vi "14_StartStop_UI.vi"(8 "error in (no error)":errorcluster) -> (0 "error out":errorcluster)   [LabVIEW 2014]
uses:
  SwabianInstruments.TimeTagger
panel:
  in  "clear":bool
  in  "binwidth":i64=1
  in  "Test signal":bool
  in  "Start channel":i32=2
  in  "Stop channel":i32=1
  in  "stop":bool
  out "StartStop Histogram":cluster{i64[], i64[]}(graph)
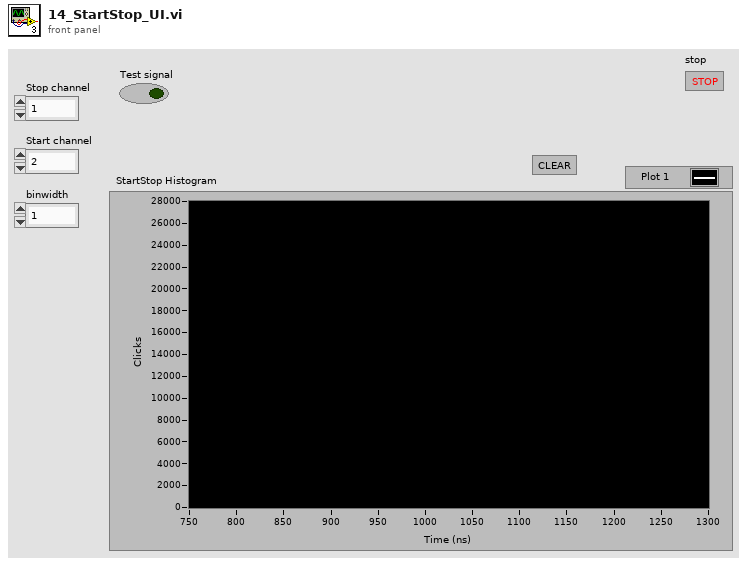
[diagram p1: front panel]
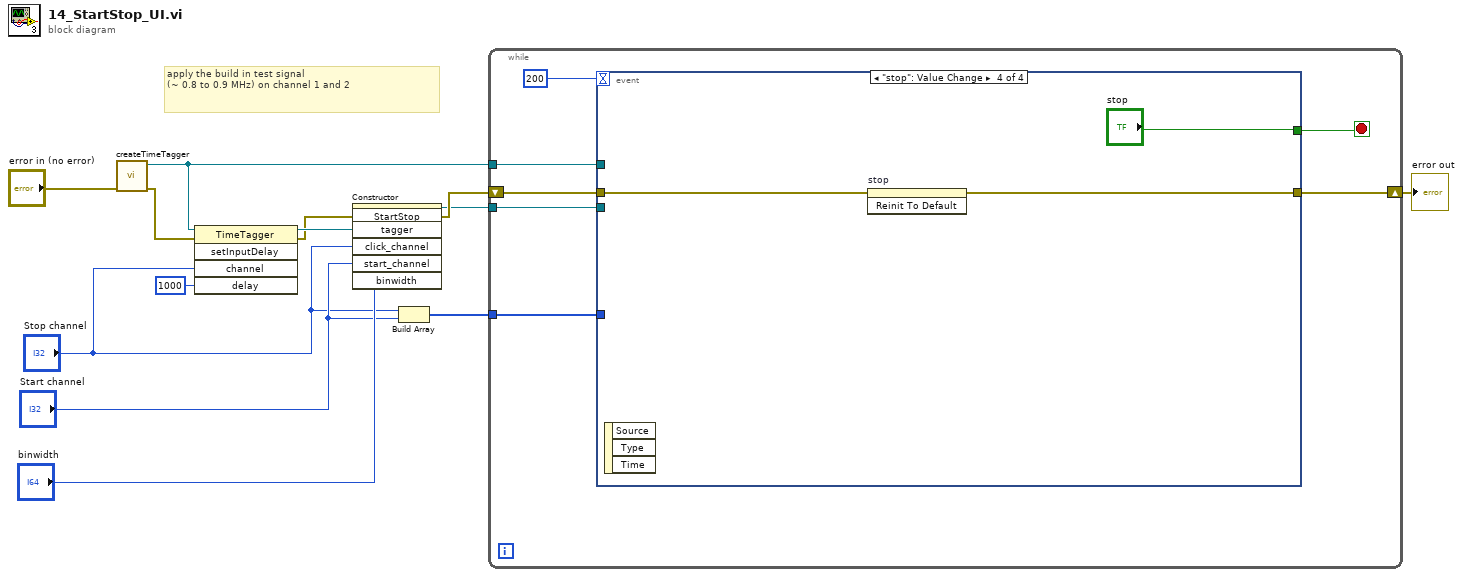
[diagram p0: block diagram]
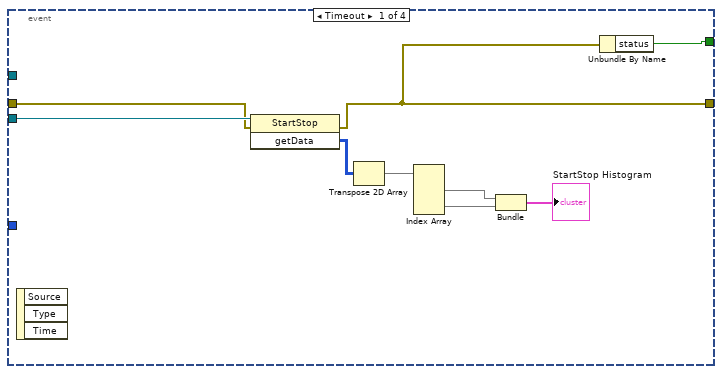
[diagram p2: hidden frame]
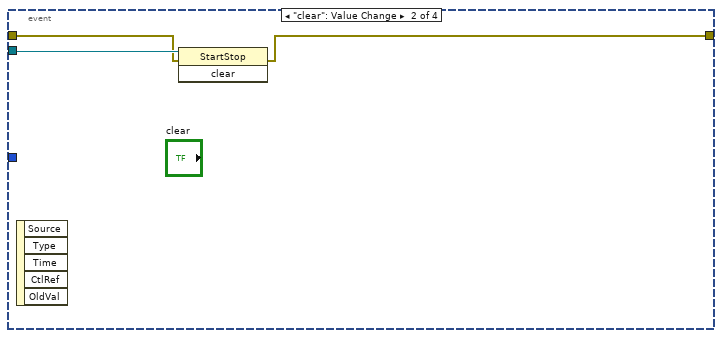
[diagram p3: hidden frame]
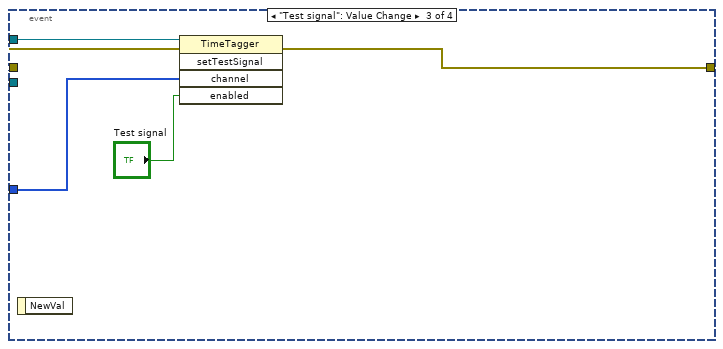
[diagram p4: hidden frame]
diagram:
  # "apply the build in test signal\n(~ 0.8 to 0.9 MHz) on channel 1 and 2"
  n1 = call "createTimeTagger.vi"("error in (no error)"="error in (no error)") -> ("error out"=w3:errorcluster, "TimeTagger ref out"=w6:refnum<k24>)  [unwired: 9 in]
  n2 = invoke class="TimeTagger" method="setInputDelay"(reference=w6, error in=w3, "channel"="Stop channel", "delay"=i64 1000) -> (reference out=w5:refnum<k24>, error out=w2:errorcluster)  [unwired: 1 in, 3 out]
  n3 = constructor class="StartStop"(error in=w2, "tagger"=w5, "click_channel"="Stop channel", "start_channel"="Start channel", "binwidth"="binwidth") -> (reference out=w12:refnum<k24>, error out=w13:errorcluster)  [unwired: 2 in, 5 out]
  n4 = Build Array("Stop channel", "Start channel") -> (w9:i32[])
  n5 = while {
    tunnel: w6 -> [w19]
    shift-right: [w18] -> w7
    shift-left: w13 -> [w20]
    tunnel: w12 -> [w17]
    tunnel: w9 -> [w15]
    stop <- w14 stop-if-true
    n6 = event shown="[3] \"stop\": Value Change" {
      selector: _ -> [_ _ _ _]
      dyn-events: _ -> [_ _ _ _]
      timeout: 200 -> [_ _ _ _]
      tunnel: w20 -> [w27 w31 w36 w39]
      tunnel: w19 -> [_ _ w37 _]
      tunnel: [w22 w30 w33 w38] -> w18
      tunnel: w17 -> [w28 w32 _ _]
      tunnel: w15 -> [_ _ w34 _]
      tunnel: [w21 _ _ "stop"] -> w14
      event Timeout {
        n7 = event-data() -> ()  [unwired: 1 in, 3 out]
        n8 = invoke class="StartStop" method="getData"(reference=w28, error in=w27) -> (error out=w22:errorcluster, "getData"=w24:i64[][])  [unwired: 1 in, 1 out]
        n9 = Transpose 2D Array(2D array=w24) -> (transposed array=w23:i64[][])
        n10 = Index Array(array=w23) -> (element #1=w26:i64[], element #2=w25:i64[])  [unwired: 4 in]
        n11 = Bundle(w26, w25) -> (→"StartStop Histogram":cluster{i64[], i64[]})  [unwired: 1 in]
        n12 = Unbundle By Name(w22) -> ("status"=w21:bool)
      }
      event "clear": Value Change {
        n13 = event-data() -> ()  [unwired: 1 in, 5 out]
        n14 = invoke class="StartStop" method="clear"(reference=w32, error in=w31) -> (error out=w30:errorcluster)  [unwired: 1 in, 2 out]
      }
      event "Test signal": Value Change {
        n15 = event-data() -> ()  [unwired: 1 in, 1 out]
        n16 = invoke class="TimeTagger" method="setTestSignal"(reference=w37, error in=w36, "channel"=w34, "enabled"="Test signal") -> (error out=w33:errorcluster)  [unwired: 1 in, 4 out]
      }
      event "stop": Value Change {
        n17 = event-data() -> ()  [unwired: 1 in, 3 out]
        n18 = invoke on="stop" class="Bool (strict)" method="Reinit To Default"(error in=w39) -> (error out=w38:errorcluster)  [unwired: 2 in, 2 out]
      }
    }
  }
  "error out" <- w7
